vi "Move.vi"(8 "error in (no error)":errorcluster, 9 "New path":string, 10 "Path":string, 11 "File Transfer Behavior in":refnum<class "File Transfer Behavior.lvclass">) -> (0 "error out":errorcluster, 3 "File Transfer Behavior out":refnum<class "File Transfer Behavior.lvclass">)   [LabVIEW 2015, in "RT Management.lvlib" / "File Transfer Behavior.lvclass"]
doc: "Moves the file located at \"Path\" to \"New path\". The VI also creates all needed directories if the \"New path\" contains directories that don't exist on the target.\n\nThe recommended file path format for \"Remote path\" is \"/directory1/directory2/file.extension\". However, the VI will accept other formats and transform the path appropriately in most cases. Use the \"Strip path.vi\" and \"Build path.vi\" VIs to help with handling remote path strings."
uses:
  File Transfer Behavior.lvclass
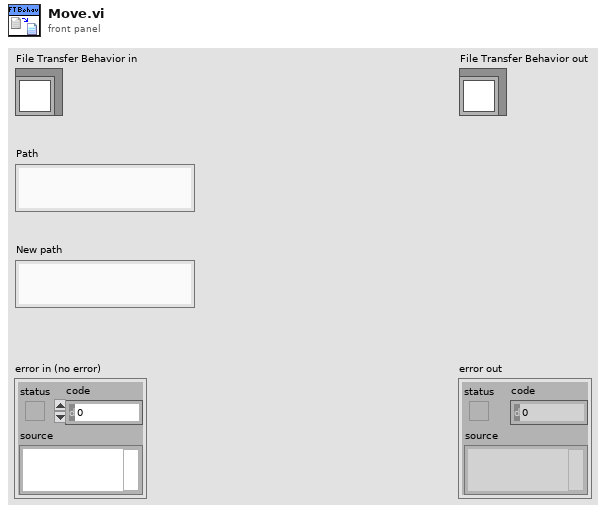
[diagram p1: front panel]
types:
  T1 = typedef "RT Management.lvlib/File Transfer Behavior.lvclass/Type.ctl" = enum16{"unknown", "file", "directory"}
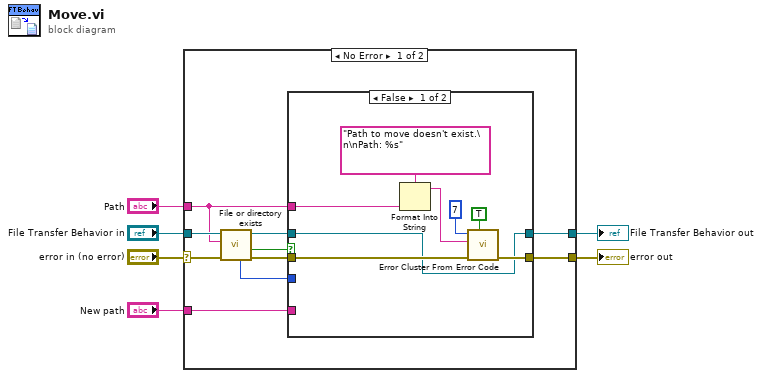
[diagram p0: block diagram]
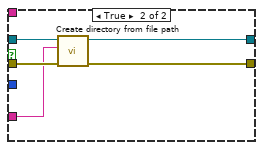
[diagram p2: hidden frame]
diagram:
  n1 = case shown="No Error" "error in (no error)" {
    selector: "error in (no error)" -> [w16 w31]
    tunnel: [w12 w31] -> w5
    tunnel: [w7 w30] -> w3
    tunnel: "File Transfer Behavior in" -> [w15 w30]
    tunnel: "Path" -> [w11 _]
    tunnel: "New path" -> [w9 _]
    frame No Error {
      n2 = call-dynamic "File or directory exists.vi"("error in (no error)"=w16, "Path"=w11, "File Transfer Behavior in"=w15) -> ("error out"=w14:errorcluster, "Exists?"=w13:bool, "File Transfer Behavior out"=w8:refnum<class "File Transfer Behavior.lvclass">, "Type"=w10:T1)  [unwired: 4 in, 1 out]
      n3 = case shown="False" w13 {
        tunnel: w14 -> [w24 w29]
        tunnel: [w23 w26] -> w12
        tunnel: w11 -> [w18 _]
        tunnel: w10 -> [_ _]
        tunnel: w8 -> [w17 w28]
        tunnel: w9 -> [_ w27]
        tunnel: [w17 w25] -> w7
        frame False {
          n4 = Format Into String(format string="Path to move doesn't exist.\n\nPath: %s" ("error message (\"\")"), w18) -> (resulting string=w19:string)  [unwired: 2 in, 1 out]
          n5 = call <vilib>:"Error Cluster From Error Code.vi"("show call chain? (False)"=TRUE, "error in (no error)"=w24, "error message (\"\")"=w19, "error code (0)"=7) -> ("error out"=w23:errorcluster)  [unwired: 5 in]
        }
        frame True {
          n6 = call "Create directory from file path.vi"("error in (no error)"=w29, "File path"=w27, "File Transfer Behavior in"=w28) -> ("error out"=w26:errorcluster, "File Transfer Behavior out"=w25:refnum<class "File Transfer Behavior.lvclass">)  [unwired: 7 in]
        }
      }
    }
    frame Error {
    }
  }
  "error out" <- w5
  "File Transfer Behavior out" <- w3
